vi "Clamp Horizontal Max VI.vi"(0 "Image":T3, 2 "Rectangle":T5 {"Rotation" format="%.2f"; "Left" scale=0.0..1024.0; "Right" scale=0.0..1024.0}, 3 "Coordinate System":T4 {"Measurement System"."Axis Reference" items=["Direct", "Indirect"]; "Measurement System"."Angle (deg)" format="%.2f"; "Measurement System"."Origin"."Y" format="%.2f"; "Measurement System"."Origin"."X" format="%.2f"; "Reference System"."Axis Reference" items=["Direct", "Indirect"]; "Reference System"."Angle (deg)" format="%.2f"; "Reference System"."Origin"."Y" format="%.2f"; "Reference System"."Origin"."X" format="%.2f"}, 5 "error in (no error)":errorcluster, 8 "Settings":T2={"Contrast"=40, "Filter width"=4, "Steepness"=2, "Subsampling Ratio"=5, "Show Search Area"=FALSE, "Show Search Lines"=FALSE, "Show Edges Found"=FALSE, "Show Result"=TRUE}) -> (7 "Line Coordinates":T1(array[cluster]) {"?"."Y" format="%.2f"; "?"."X" format="%.2f"; "?"."Y" format="%.2f"; "?"."X" format="%.2f"}, 9 "appended array":cluster{"X":sgl, "Y":sgl}[](array[cluster]), 10 "Edge Coordinates":cluster{"X":sgl, "Y":sgl}[](array[cluster]) {"Y" format="%.2f"; "X" format="%.2f"}, 11 "Perpendicular Lines":T1(array[cluster])=[{{"X"=55.0, "Y"=48.0}, {"X"=263.0, "Y"=104.0}}, {{"X"=53.0, "Y"=53.0}, {"X"=262.0, "Y"=109.0}}, {{"X"=52.0, "Y"=58.0}, {"X"=261.0, "Y"=113.0}}, {{"X"=51.0, "Y"=62.0}, {"X"=259.0, "Y"=118.0}}, {{"X"=49.0, "Y"=67.0}, {"X"=258.0, "Y"=123.0}}, {{"X"=48.0, "Y"=72.0}, {"X"=257.0, "Y"=128.0}}, {{"X"=47.0, "Y"=77.0}, {"X"=255.0, "Y"=133.0}}, {{"X"=46.0, "Y"=82.0}, {"X"=254.0, "Y"=138.0}}, {{"X"=44.0, "Y"=87.0}, {"X"=253.0, "Y"=142.0}}, {{"X"=43.0, "Y"=91.0}, {"X"=252.0, "Y"=147.0}}, {{"X"=42.0, "Y"=96.0}, {"X"=250.0, "Y"=152.0}}] {"?"."Y" format="%.2f"; "?"."X" format="%.2f"; "?"."Y" format="%.2f"; "?"."X" format="%.2f"}, 13 "Points":cluster{"X":sgl, "Y":sgl}[](array[cluster])=[{"X"=67.0, "Y"=51.0}, {"X"=230.0, "Y"=95.0}, {"X"=66.0, "Y"=56.0}, {"X"=230.0, "Y"=100.0}, {"X"=66.0, "Y"=62.0}, {"X"=230.0, "Y"=105.0}, {"X"=66.0, "Y"=66.0}, {"X"=230.0, "Y"=110.0}, {"X"=65.0, "Y"=71.0}, {"X"=230.0, "Y"=115.0}, {"X"=65.0, "Y"=77.0}, {"X"=230.0, "Y"=121.0}, {"X"=65.0, "Y"=82.0}, {"X"=229.0, "Y"=126.0}, {"X"=65.0, "Y"=87.0}, {"X"=229.0, "Y"=131.0}, {"X"=64.0, "Y"=92.0}, {"X"=229.0, "Y"=136.0}, {"X"=64.0, "Y"=97.0}, {"X"=229.0, "Y"=141.0}, {"X"=64.0, "Y"=102.0}, {"X"=229.0, "Y"=146.0}] {"Y" format="%.2f"; "X" format="%.2f"}, 14 "Image Out":T3, 16 "Distance":sgl format="%.2f", 17 "Coordinate System (duplicate)":T4 {"Measurement System"."Axis Reference" items=["Direct", "Indirect"]; "Measurement System"."Angle (deg)" format="%.2f"; "Measurement System"."Origin"."Y" format="%.2f"; "Measurement System"."Origin"."X" format="%.2f"; "Reference System"."Axis Reference" items=["Direct", "Indirect"]; "Reference System"."Angle (deg)" format="%.2f"; "Reference System"."Origin"."Y" format="%.2f"; "Reference System"."Origin"."X" format="%.2f"}, 19 "error out":errorcluster)   [LabVIEW 2019]
uses:
  <vilib>/vision/Image Controls.llb/IMAQ Image.ctl
  <vilib>/vision/NI_Vision_Development_Module.lvlib
panel:
  out "Elapsed time (ms)":u32
  # "Start Point"
  # "End Point"
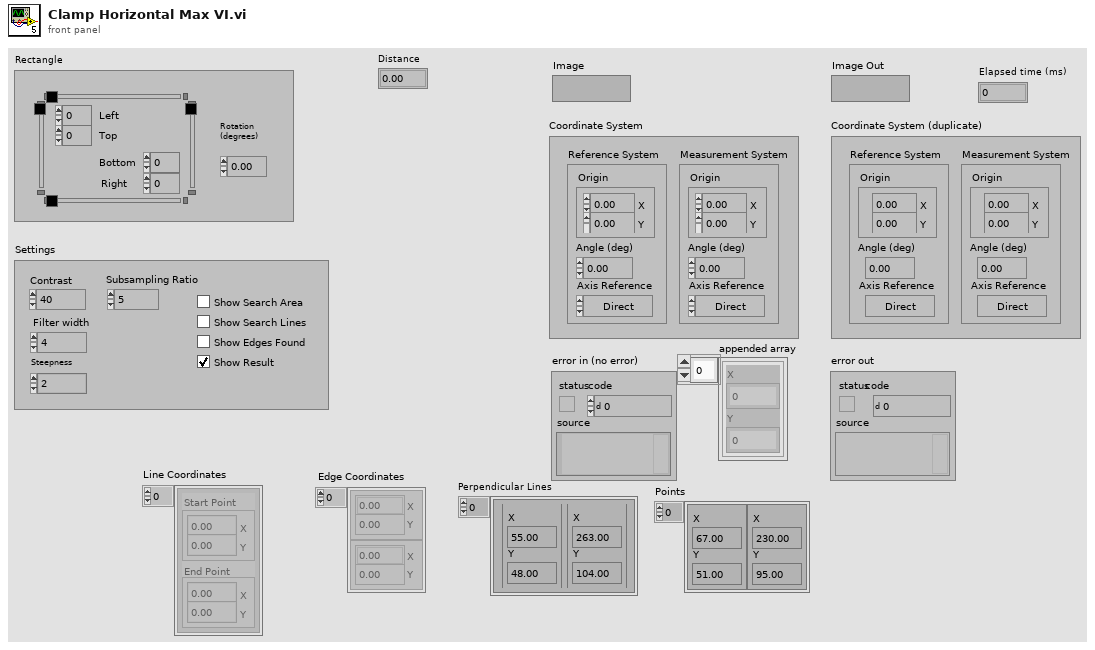
[diagram p1: front panel]
types:
  T1 = cluster{cluster{"X":sgl, "Y":sgl}, cluster{"X":sgl, "Y":sgl}}[]
  T2 = cluster{"Contrast":i32, "Filter width":i32, "Steepness":i32, "Subsampling Ratio":u32, "Show Search Area":bool, "Show Search Lines":bool, "Show Edges Found":bool, "Show Result":bool}
  T3 = typedef "IMAQ Image.ctl" = refnum<image>
  T4 = typedef "IMAQ Coordinate System" = cluster{"Reference System":cluster{"Origin":cluster{"X":sgl, "Y":sgl}, "Angle (deg)":sgl, "Axis Reference":u32}, "Measurement System":cluster{"Origin":cluster{"X":sgl, "Y":sgl}, "Angle (deg)":sgl, "Axis Reference":u32}}
  T5 = typedef "IMAQ Rectangle" = cluster{"Left":i32, "Top":i32, "Right":i32, "Bottom":i32, "Rotation":dbl}
  T6 = cluster{"Interpolation Type":enum32{"", "Quadratic", "Cubic Spline"}, "SubPixel Accuracy":enum32{"None", "One Half", "One Third", "One Fourth", "One Fifth", "One Sixth", "One Seventh", "One Eight", "One Ninth", "One Tenth", "One Eleventh", "One Twelveth"}}
  T7 = enum32{"Get First Edge", "Get First + Last Edge", "Get All Edges"}
  T8 = cluster{"Origin":cluster{"X":sgl, "Y":sgl}, "Angle (deg)":sgl, "Axis Reference":u32}
  T9 = typedef "ROI Descriptor" = cluster{"Global Rectangle":i32[], "Contours":cluster{"ID":enum32{"External", "Internal"}, "Type":u32, "Coordinates":i32[]}[]}
  T10 = cluster{"Contrast":i32, "Filter width":i32, "Steepness":i32}
  T11 = cluster{"Show Search Area":bool, "Show Search Lines":bool, "Show Edges Found":bool, "Show Result":bool}
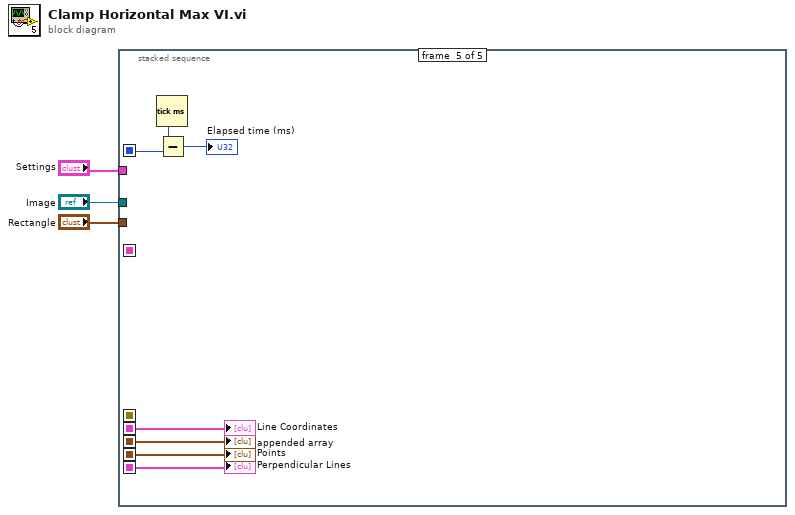
[diagram p0: block diagram]
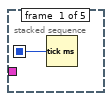
[diagram p2: hidden frame]
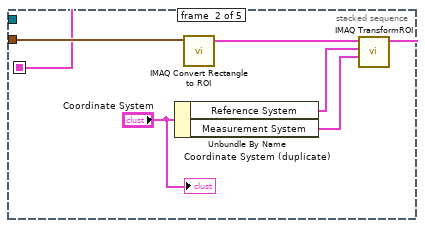
[diagram p3: hidden frame]
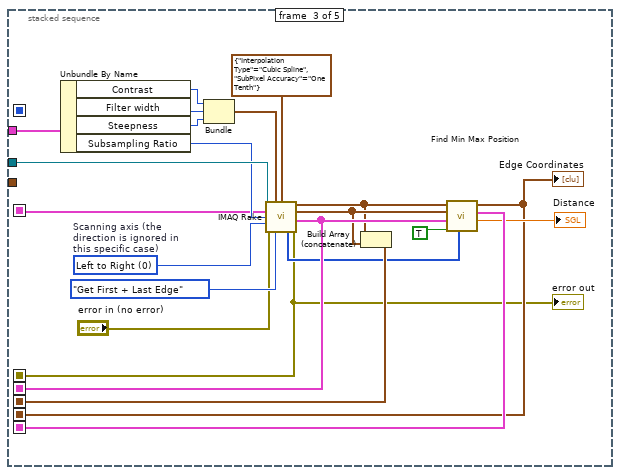
[diagram p4: hidden frame]
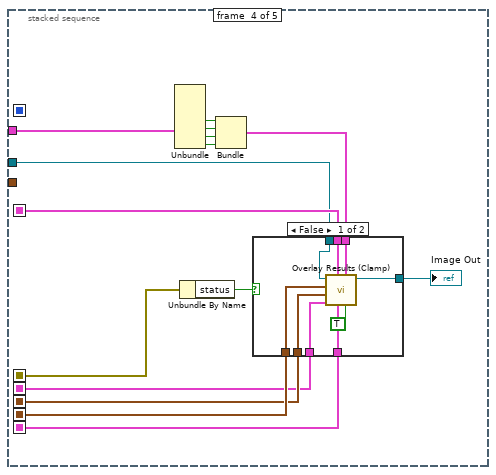
[diagram p5: hidden frame]
diagram:
  n1 = stacked-sequence {
    seq-local: [_ _ w23 _ _] -> [_ _ _ w47 w59]
    seq-local: [w4 _ _ _ _] -> [_ _ _ _ w64]
    seq-local: [_ _ w18 _ _] -> [_ _ _ w46 w60]
    seq-local: [_ _ w21 _ _] -> [_ _ _ w33 w61]
    seq-local: [_ _ w25 _ _] -> [_ _ _ w40 w58]
    seq-local: [_ w7 _ _ _] -> [_ _ w13 w38 _]
    seq-local: [_ _ w11 _ _] -> [_ _ _ w35 _]
    tunnel: "Image" -> [_ _ w27 w34 _]
    tunnel: "Rectangle" -> [_ w8 _ _ _]
    tunnel: "Settings" -> [_ _ w26 w45 _]
    frame #0 {
      n2 = Tick Count (ms)() -> (millisecond timer value=w4:u32)
    }
    frame #1 {
      n3 = Unbundle By Name("Coordinate System") -> ("Reference System"=w6:T8, "Measurement System"=w5:T8)
      n4 = call "IMAQ Convert Rectangle to ROI"("Rectangle"=w8) -> ("ROI Descriptor"=w10:T9)  [unwired: 1 in, 8 out]
      n5 = call "IMAQ TransformROI"("New Reference"=w5, "Base Reference"=w6, "ROI Descriptor"=w10) -> ("ROI Descriptor out"=w7:T9)  [unwired: 1 in, 7 out]
      "Coordinate System (duplicate)" <- "Coordinate System"
    }
    frame #2 {
      w28 = u32 0 items=["Left to Right", "Right to Left", "Top to Bottom", "Bottom to Top"]  # Scanning axis (the direction is ignored in this specific case)
      # "Find Edges"
      n6 = Unbundle By Name(w26) -> ("Contrast"=w17:i32, "Filter width"=w16:i32, "Steepness"=w15:i32, "Subsampling Ratio"=w14:u32)
      n7 = Bundle("Contrast"=w17, "Filter width"=w16, "Steepness"=w15) -> (w32:T10)  [unwired: 1 out]
      n8 = call "IMAQ Rake"("Image"=w27, "Edge Parameters"=w32, "SubPixel Information"=T6 {"Interpolation Type"=enum."Cubic Spline", "SubPixel Accuracy"=enum."One Tenth"}, "ROI Descriptor"=w13, "Step Size"=w14, "Scan Direction"=w28, "error in (no error)"="error in (no error)", "Process"=T7."Get First + Last Edge") -> ("First Edges"=w19:cluster{"X":sgl, "Y":sgl}[], "Last Edges"=w20:cluster{"X":sgl, "Y":sgl}[], "Line Coordinates"=w21:T1, "Lines with Edges"=w12:u32[], "error out"=w11:errorcluster)  [unwired: 1 in, 2 out]
      "error out" <- w11
      n9 = Build Array (concatenate)(w19, w20) -> (w18:cluster{"X":sgl, "Y":sgl}[])
      n10 = call <vilib>:"Find Min Max Position.vi"("Lines with Edges (first)"=w12, "Min / Max"=TRUE, "Search Lines"=w21, "Last Edges"=w20, "First Edges"=w19) -> ("Distance"=→"Distance":sgl, "Perpendicular Lines"=w25:T1, "Points"=w23:cluster{"X":sgl, "Y":sgl}[])  [unwired: 1 in, 3 out]
      "Edge Coordinates" <- w23
    }
    frame #3 {
      # "Update Overlay"
      n11 = Unbundle(w45) -> ("Show Search Area"=w44:bool, "Show Search Lines"=w43:bool, "Show Edges Found"=w42:bool, "Show Result"=w41:bool)  [unwired: 4 out]
      n12 = Unbundle By Name(w35) -> ("status"=w36:bool)
      n13 = Bundle("Show Search Area"=w44, "Show Search Lines"=w43, "Show Edges Found"=w42, "Show Result"=w41) -> (w39:T11)  [unwired: 1 out]
      n14 = case shown="False" w36 {
        tunnel: w47 -> [w56 _]
        tunnel: w46 -> [w55 _]
        tunnel: w33 -> [w54 _]
        tunnel: w40 -> [w53 _]
        tunnel: w39 -> [w51 _]
        tunnel: w38 -> [w50 _]
        tunnel: w34 -> [w48 w57]
        tunnel: [w49 w57] -> w37
        frame False {
          n15 = call <vilib>:"Overlay Results (Clamp).vi"("Min / Max"=TRUE, "Setup"=w51, "Perpendicular Lines"=w53, "ROI Descriptor"=w50, "Search Lines"=w54, "All Edges Found"=w55, "Measurement Edges"=w56, "Image In"=w48) -> ("Image Out"=w49:T3)  [unwired: 3 out]
        }
        frame True {
        }
      }
      "Image Out" <- w37
    }
    frame #4 {
      n16 = Tick Count (ms)() -> (millisecond timer value=w63:u32)
      n17 = Subtract(x=w63, y=w64) -> (x-y=→"Elapsed time (ms)":u32)
      "Line Coordinates" <- w61
      "appended array" <- w60
      "Points" <- w59
      "Perpendicular Lines" <- w58
    }
  }
